vi "main.vi"() -> ()   [LabVIEW 2017]
panel:
  in  "millisecond multiple":u32=5
  in  "s":sgl=5.0
  in  "MULTI":bool
  out "max value":u32
  out "Array":u32[](array[numeric])
  in  "a/d":sgl=0.1
  in  "V":sgl=0.1
  in  "p":sgl=-10.0
  out "NIBBLE":i32
  out "Enable":bool
  in  "GOTO":bool
  in  "DISABLE":bool
  in  "ENABLE":bool
  in  "Curve":bool
  out "Connected":bool
  in  "DISCONNECT":bool
  in  "Connect":bool
  out "Working":bool
  in  "ACK":bool
  in  "HOME":bool
  in  "G_Enable":bool
  in  "OPERATIONAL":bool
  in  "stop":bool
  out "error out":errorcluster
  in  "error in (no error)":errorcluster
  in  "VISA resource name":refnum<visa-resource-name>
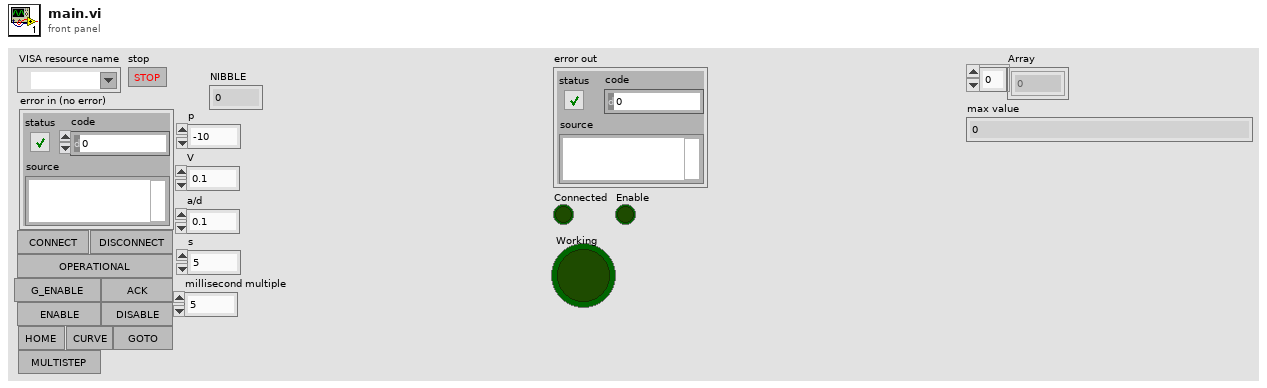
[diagram p1: front panel]
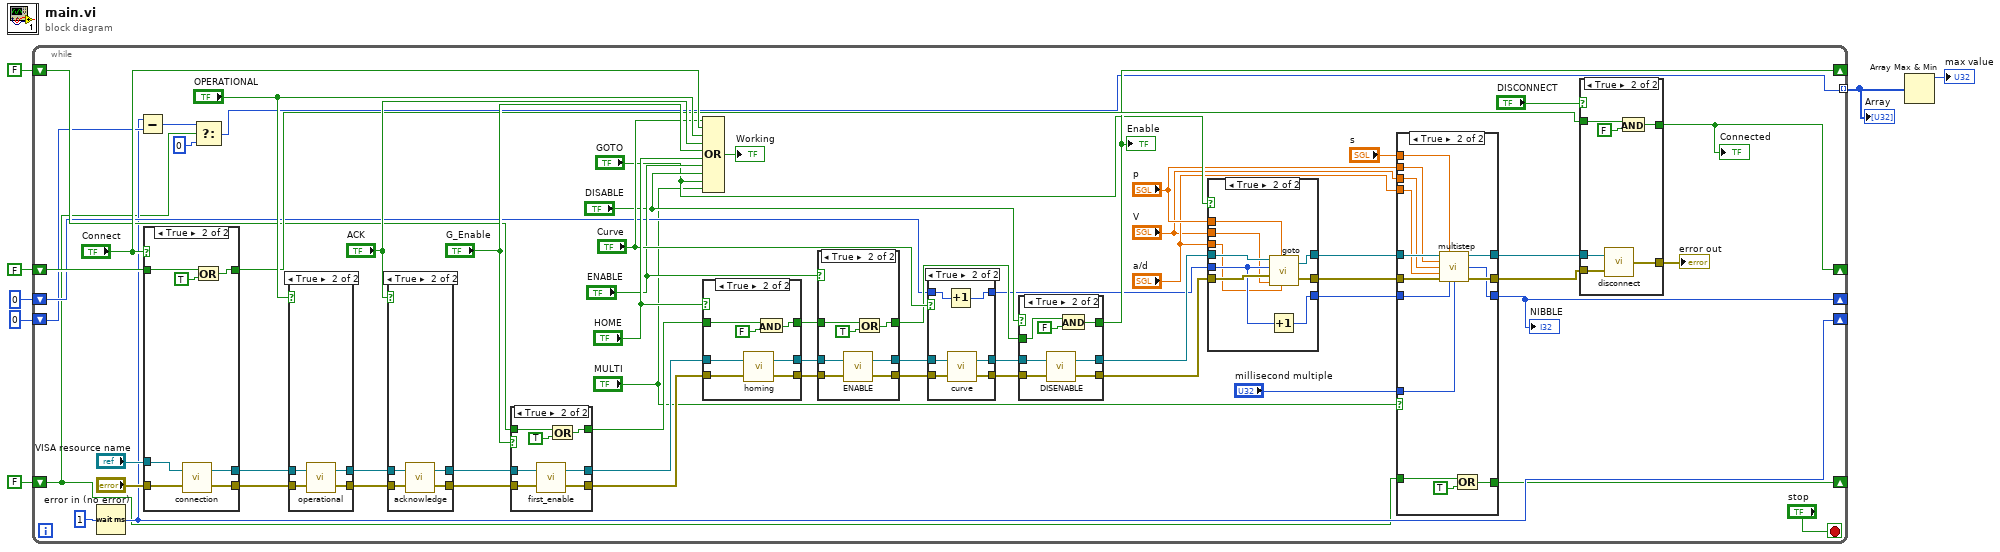
[diagram p0: block diagram]
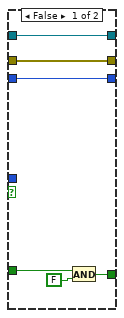
[diagram p2: hidden frame]
diagram:
  n1 = while {
    shift-right: [w47] -> _
    shift-left: FALSE -> [w49]
    shift-right: [w33] -> _
    shift-left: FALSE -> [w35]
    shift-right: [w13] -> _
    shift-left: 0 -> [w30]
    tunnel: [w26] -> w3 mode=indexing
    shift-right: [w23] -> _
    shift-left: 0 -> [w24]
    shift-right: [w9] -> _
    shift-left: FALSE -> [w10]
    stop <- "stop" stop-if-true
    n2 = Wait (ms)(milliseconds to wait=u32 1 ("millisecond multiple")) -> (millisecond timer value=w23:u32)
    n3 = Subtract(x=w23, y=w24) -> (x-y=w22:u32)
    n4 = case shown="True" "Connect" {
      tunnel: "VISA resource name" -> [w138 w147]
      tunnel: "error in (no error)" -> [w139 w146]
      tunnel: [w139 w145] -> w53
      tunnel: [w138 w144] -> w52
      tunnel: w49 -> [w140 w143]
      tunnel: [w140 w141] -> w48
      frame False {
      }
      frame True {
        n5 = call "connection.vi"("error out"=w146, "VISA resource name"=w147) -> ("error out 2"=w145:errorcluster, "VISA resource name 2"=w144:refnum<visa-resource-name>)
        n6 = Or(x=w143, y=TRUE) -> (x .or. y?=w141:bool)
      }
    }
    n7 = Select(t=w22, s=w10, f=0) -> (s? t:f=w26:u32)
    n8 = case shown="True" "OPERATIONAL" {
      tunnel: w52 -> [w155 w159]
      tunnel: [w155 w158] -> w65
      tunnel: [w154 w157] -> w62
      tunnel: w53 -> [w154 w156]
      frame False {
      }
      frame True {
        n9 = call "operational.vi"("error out 4"=w156, "VISA resource name 4"=w159) -> ("error out 5"=w157:errorcluster, "VISA resource name 5"=w158:refnum<visa-resource-name>)
      }
    }
    n10 = case shown="True" "ACK" {
      tunnel: w65 -> [w149 w153]
      tunnel: [w149 w152] -> w64
      tunnel: [w148 w151] -> w63
      tunnel: w62 -> [w148 w150]
      frame False {
      }
      frame True {
        n11 = call "acknowledge.vi"("error out 4"=w150, "VISA resource name 4"=w153) -> ("error out 5"=w151:errorcluster, "VISA resource name 5"=w152:refnum<visa-resource-name>)
      }
    }
    n12 = case shown="True" "G_Enable" {
      tunnel: [w172 w179] -> w68
      tunnel: [w171 w178] -> w67
      tunnel: w63 -> [w171 w177]
      tunnel: w64 -> [w172 w176]
      tunnel: w35 -> [w170 w174]
      tunnel: [w170 w173] -> w32
      frame False {
      }
      frame True {
        n13 = call "first_enable.vi"("error out 2"=w177, "VISA resource name 2"=w176) -> ("error out 3"=w178:errorcluster, "VISA resource name 3"=w179:refnum<visa-resource-name>)
        n14 = Or(x=w174, y=TRUE) -> (x .or. y?=w173:bool)
      }
    }
    n15 = Compound Arithmetic op=OR("Curve", "Connect", "OPERATIONAL", "ACK", "G_Enable", "HOME", "ENABLE", "DISABLE", "GOTO", "MULTI") -> (→"Working":bool)
    n16 = case shown="True" "HOME" {
      tunnel: [w162 w167] -> w42
      tunnel: [w161 w166] -> w43
      tunnel: w68 -> [w162 w169]
      tunnel: w67 -> [w161 w168]
      tunnel: w32 -> [w160 w164]
      tunnel: [w160 w163] -> w31
      frame False {
      }
      frame True {
        n17 = call "homing.vi"("error out 4"=w168, "VISA resource name 4"=w169) -> ("error out 5"=w166:errorcluster, "VISA resource name 5"=w167:refnum<visa-resource-name>)
        n18 = And(x=w164, y=FALSE) -> (x .and. y?=w163:bool)
      }
    }
    n19 = case shown="True" "ENABLE" {
      tunnel: [w112 w120] -> w45
      tunnel: [w113 w119] -> w44
      tunnel: w43 -> [w112 w118]
      tunnel: w42 -> [w113 w117]
      tunnel: w31 -> [w111 w115]
      tunnel: [w111 w114] -> w34
      frame False {
      }
      frame True {
        n20 = call "ENABLE.vi"("error out 4"=w118, "VISA resource name 4"=w117) -> ("error out 5"=w120:errorcluster, "VISA resource name 5"=w119:refnum<visa-resource-name>)
        n21 = Or(x=w115, y=TRUE) -> (x .or. y?=w114:bool)
      }
    }
    n22 = case shown="True" "Curve" {
      tunnel: w44 -> [w123 w129]
      tunnel: w45 -> [w122 w128]
      tunnel: [w123 w127] -> w41
      tunnel: [w122 w126] -> w40
      tunnel: w30 -> [w121 w125]
      tunnel: [w121 w124] -> w29
      frame False {
      }
      frame True {
        n23 = Increment(x=w125) -> (x+1=w124:i32)
        n24 = call "curve.vi"("error out 4"=w128, "VISA resource name 4"=w129) -> ("error out 5"=w126:errorcluster, "VISA resource name 5"=w127:refnum<visa-resource-name>)
      }
    }
    n25 = case shown="True" "DISABLE" {
      tunnel: w41 -> [w103 w110]
      tunnel: w40 -> [w102 w109]
      tunnel: [w103 w108] -> w37
      tunnel: [w102 w107] -> w36
      tunnel: w34 -> [w101 w105]
      tunnel: [w101 w104] -> w33
      frame False {
      }
      frame True {
        n26 = call "DISENABLE.vi"("error out 4"=w109, "VISA resource name 4"=w110) -> ("error out 5"=w107:errorcluster, "VISA resource name 5"=w108:refnum<visa-resource-name>)
        n27 = And(x=w105, y=FALSE) -> (x .and. y?=w104:bool)
      }
    }
    "Enable" <- w33
    n28 = case shown="True" "GOTO" {
      tunnel: w37 -> [w91 w100]
      tunnel: w36 -> [w90 w99]
      tunnel: [w91 w98] -> w21
      tunnel: [w90 w97] -> w19
      tunnel: w29 -> [w89 w96]
      tunnel: [w89 w95] -> w14
      tunnel: "p" -> [_ w94]
      tunnel: "V" -> [_ w93]
      tunnel: "a/d" -> [_ w92]
      frame False {
      }
      frame True {
        n29 = Increment(x=w96) -> (x+1=w95:i32)
        n30 = call "goto.vi"("Numeric 3"=w92, "Numeric"=w94, "Numeric 2"=w93, "error out 2"=w99, "new element/subarray"=w96, "VISA resource name 2"=w100) -> ("error out 3"=w97:errorcluster, "VISA resource name 3"=w98:refnum<visa-resource-name>)
      }
    }
    n31 = case shown="True" "MULTI" {
      tunnel: w21 -> [w73 w88]
      tunnel: [w73 w87] -> w20
      tunnel: w19 -> [w72 w85]
      tunnel: [w72 w86] -> w18
      tunnel: "p" -> [_ w83]
      tunnel: "a/d" -> [_ w82]
      tunnel: "V" -> [_ w81]
      tunnel: w14 -> [w74 w80]
      tunnel: [w74 w84] -> w13
      tunnel: "s" -> [_ w79]
      tunnel: w10 -> [w70 w77]
      tunnel: [w69 w76] -> w9
      tunnel: "millisecond multiple" -> [_ w75]
      frame False {
        n32 = And(x=w70, y=FALSE) -> (x .and. y?=w69:bool)
      }
      frame True {
        n33 = call "multistep.vi"("VISA resource name 2"=w88, "y"=w79, "Numeric 5"=w83, "Numeric 2"=w81, "Numeric 3"=w82, "error out 2"=w85, "new element/subarray"=w80, "millisecond multiple"=w75) -> ("VISA resource name 3"=w87:refnum<visa-resource-name>, "Numeric 4"=w84:i32, "error out 3"=w86:errorcluster)  [unwired: 5 in]
        n34 = Or(x=w77, y=TRUE) -> (x .or. y?=w76:bool)
      }
    }
    "NIBBLE" <- w13
    n35 = case shown="True" "DISCONNECT" {
      tunnel: w20 -> [_ w137]
      tunnel: w18 -> [w130 w136]
      tunnel: [w130 w135] -> w54
      tunnel: w48 -> [w131 w133]
      tunnel: [w131 w132] -> w47
      frame False {
      }
      frame True {
        n36 = call "disconnect.vi"("error in (no error)"=w136, "VISA resource name"=w137) -> ("error out"=w135:errorcluster)
        n37 = And(x=w133, y=FALSE) -> (x .and. y?=w132:bool)
      }
    }
    "error out" <- w54
    "Connected" <- w47
  }
  "Array" <- w3
  n38 = Array Max & Min(array=w3) -> (max value=→"max value":u32)  [unwired: 3 out]
